vi "NI VeriStand - Set Alarm Data2.vi"(8 "error in (no error)":errorcluster, 10 "Alarm Data":T1 {"Trip Value" format="%.2f"; "Delay" format="%.2f"; "Low Limit" format="%.2f"; "High Limit" format="%.2f"}, 11 "Alarm in":T2) -> (0 "error out":errorcluster, 3 "Alarm out":T2)   [LabVIEW 2020, in "NI_VS Alarm ExecutionAPI.lvlib"]
doc: "Sets high limit, low limit, corresponding procedure name, delay duration, trip value, priority, state, mode, group number, priority number, name, and full name information about the alarm you specify."
uses:
  <vilib>/NI VeriStand/Execution/Alarm/NI_VS Alarm ExecutionAPI.lvlib
  <vilib>/NI VeriStand/Execution/Alarm/AlarmAPI.ctl
  NationalInstruments.VeriStand.ClientAPI
  <vilib>/NI VeriStand/Execution/Alarm/AlarmInfo.ctl
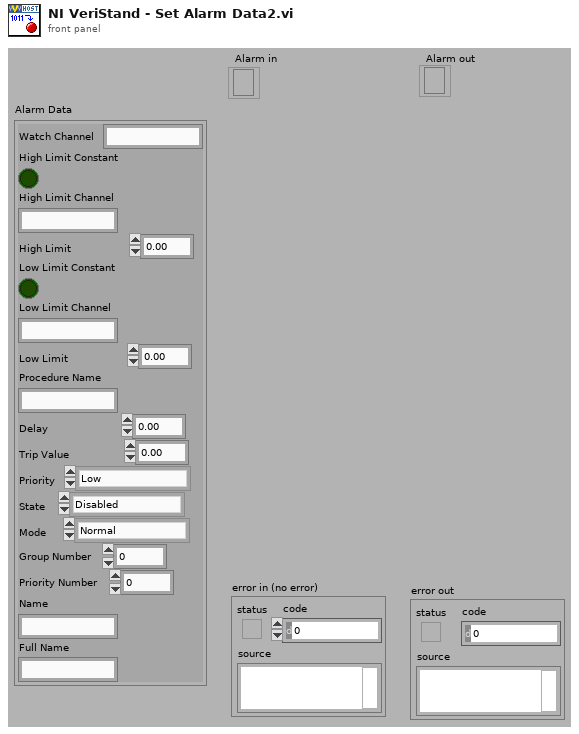
[diagram p1: front panel]
types:
  T1 = typedef "NI_VS Alarm ExecutionAPI.lvlib/AlarmInfo.ctl" = cluster{"Watch Channel":string, "High Limit Constant":bool, "High Limit Channel":string, "High Limit":dbl, "Low Limit Constant":bool, "Low Limit Channel":string, "Low Limit":dbl, "Procedure Name":string, "Delay":dbl, "Trip Value":dbl, "Priority":enum16{"Low", "Medium", "High"}, "State":enum16{"Disabled", "Enabled", "Tripped", "Delayed Trip", "Indicate"}, "Mode":enum16{"Normal", "Indicate Only"}, "Group Number":u32, "Priority Number":u32, "Name":string, "Full Name":string}
  T2 = typedef "NI_VS Alarm ExecutionAPI.lvlib/AlarmAPI.ctl" = refnum<k24>
  T3 = enum16{"Disabled", "Enabled", "Tripped", "Delayed Trip", "Indicate"}
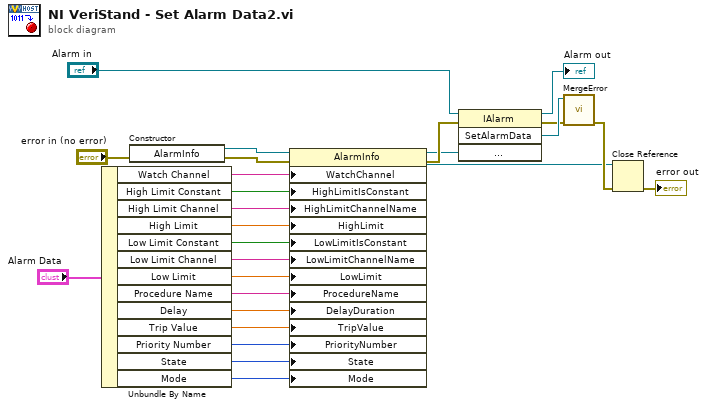
[diagram p0: block diagram]
diagram:
  n1 = Unbundle By Name("Alarm Data") -> ("Watch Channel"=w14:string, "High Limit Constant"=w13:bool, "High Limit Channel"=w12:string, "High Limit"=w11:dbl, "Low Limit Constant"=w10:bool, "Low Limit Channel"=w9:string, "Low Limit"=w8:dbl, "Procedure Name"=w7:string, "Delay"=w6:dbl, "Trip Value"=w5:dbl, "Priority Number"=w4:u32, "State"=w3:T3, "Mode"=w2:enum16{"Normal", "Indicate Only"})
  n2 = constructor class="AlarmInfo"(error in="error in (no error)") -> (reference out=w19:refnum<k24>, error out=w20:errorcluster)  [unwired: 2 in, 1 out]
  n3 = property class="AlarmInfo"(reference=w19, error in=w20, "WatchChannel"=w14, "HighLimitIsConstant"=w13, "HighLimitChannelName"=w12, "HighLimit"=w11, "LowLimitIsConstant"=w10, "LowLimitChannelName"=w9, "LowLimit"=w8, "ProcedureName"=w7, "DelayDuration"=w6, "TripValue"=w5, "PriorityNumber"=w4, "State"=w3, "Mode"=w2) -> (reference out=w1:refnum<k24>, error out=w16:errorcluster)
  n4 = invoke class="IAlarm" method="SetAlarmData"(reference="Alarm in", error in=w16, "alarmData"=w1) -> (reference out=→"Alarm out":T2, error out=w22:errorcluster, "SetAlarmData"=w23:refnum<k24>)  [unwired: 1 in, 1 out]
  n5 = call <vilib>:"MergeError.vi"("error in (no error)"=w22, "Error"=w23) -> ("error out"=w15:errorcluster)  [unwired: 9 out]
  n6 = Close Reference(reference=w1, error in (no error)=w15) -> (error out=→"error out":errorcluster)
